vi "Do.vi"(8 "error in (no error)":errorcluster, 10 "Parent Actor":refnum<class "Parent Actor.lvclass">, 11 "Toggle in":refnum<class "Toggle.lvclass">) -> (0 "error out":errorcluster, 2 "Parent Actor out":refnum<class "Parent Actor.lvclass">, 3 "Toggle out":refnum<class "Toggle.lvclass">)   [LabVIEW 2015, in "Toggle.lvclass"]
uses:
  Toggle.lvclass
  State/Parent Actor.lvclass
  Toggle.lvclass/Toggle.ctl
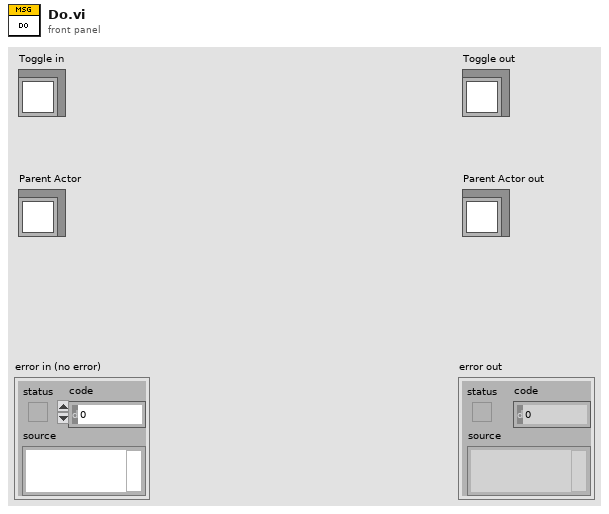
[diagram p1: front panel]
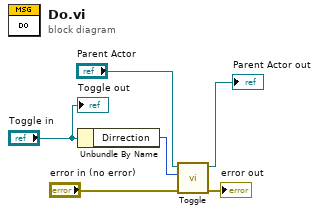
[diagram p0: block diagram]
diagram:
  n1 = Unbundle By Name("Toggle in") -> ("Dirrection"=w4:enum16{"Forward", "Reverse"})
  n2 = call-dynamic "Toggle.vi"("error in (no error)"="error in (no error)", "Dirrection"=w4, "State in"="Parent Actor") -> ("error out"=→"error out":errorcluster, "State out"=→"Parent Actor out":refnum<class "Parent Actor.lvclass">)  [unwired: 7 in]
  "Toggle out" <- "Toggle in"
